vi "writeColdCurrent.vi"(10 "Cold_current":T1) -> ()   [LabVIEW 2012]
uses:
  Cold_current.ctl
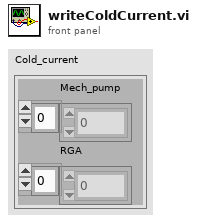
[diagram p1: front panel]
types:
  T1 = typedef "Cold_current.ctl" = cluster{"Mech_pump":i32[], "RGA":i32[]}
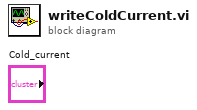
[diagram p0: block diagram]
diagram:
